vi "GET.series.vi"(4 "series offset":u32, 5 "request specific headers":T2[](array[typedef]), 6 "Number of Series to GET":u32, 7 "timeout (60000)":i32=60000, 8 "error in (no error)":errorcluster, 11 "REST Client in":refnum<class "REST Client.lvclass">) -> (0 "error out":errorcluster, 2 "data":T1, 3 "REST Client out":refnum<class "REST Client.lvclass">)   [LabVIEW 2024]
uses:
  <vilib>/addons/_JKI.lib/REST Client/classes/REST Client/HTTP Header.ctl
  <vilib>/NI/Advanced HTTP Client/Header--Combo Box.ctl
  <vilib>/addons/_JKI.lib/REST Client/classes/REST Client/REST Client.lvclass
  <vilib>/NI/Advanced HTTP Client/Session.lvclass
  TypeDefs/series.reply.ctl
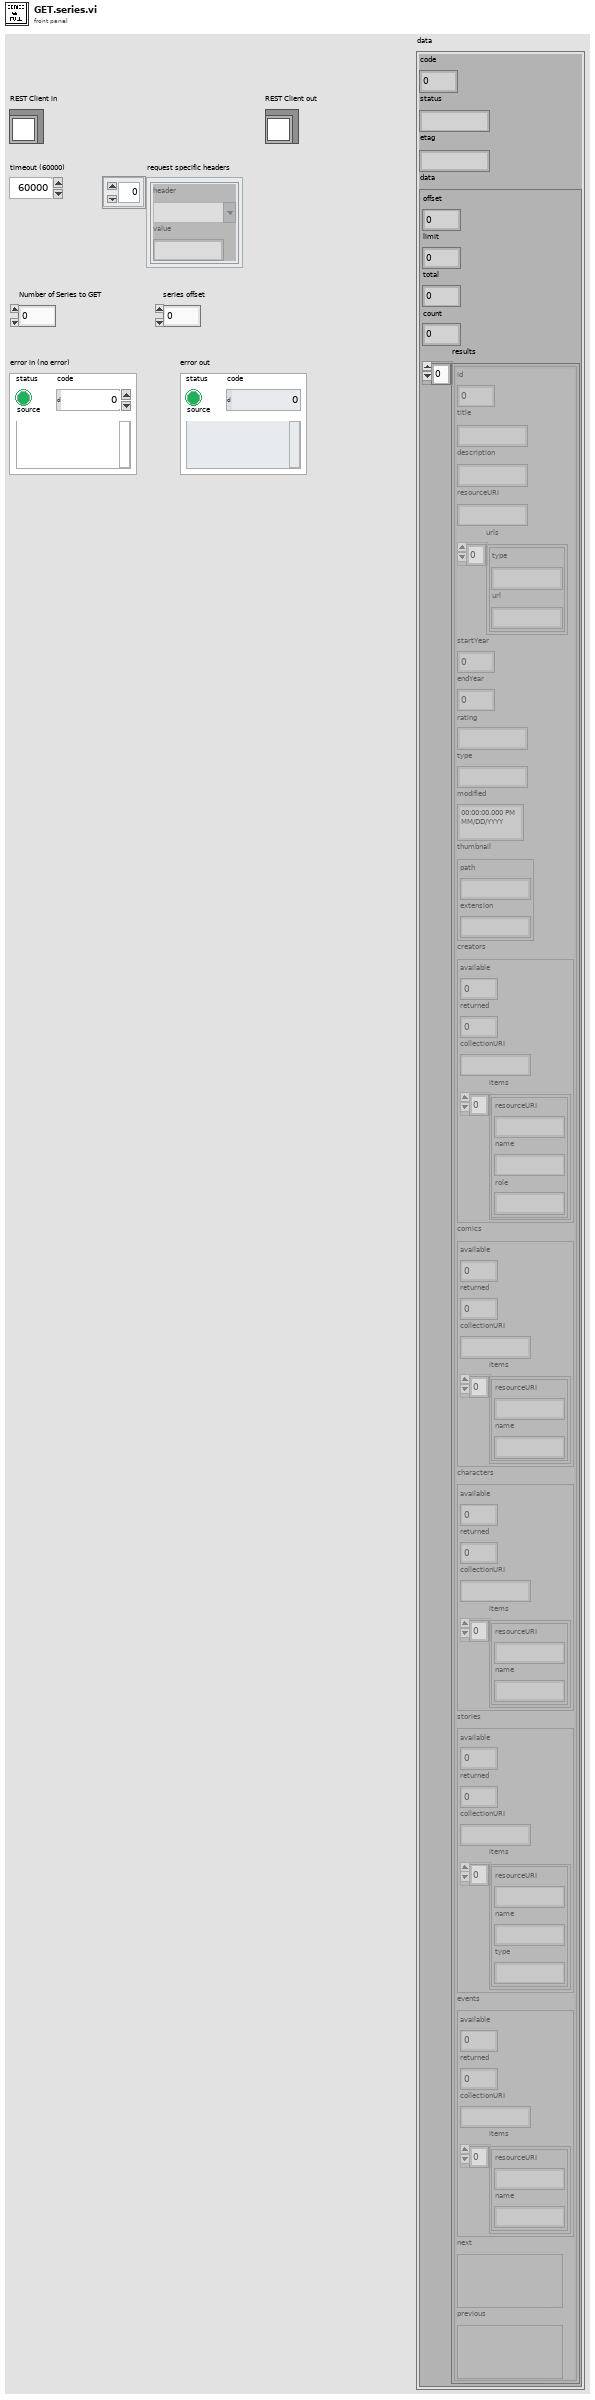
[diagram p1: front panel]
types:
  T1 = typedef "series.reply.ctl" = cluster{"code":i32, "status":string, "etag":string, "data":cluster{"offset":i32, "limit":i32, "total":i32, "count":i32, "results":cluster{"id":i32, "title":string, "description":string, "resourceURI":string, "urls":cluster{"type":string, "url":string}[], "startYear":i32, "endYear":i32, "rating":string, "type":string, "modified":timestamp, "thumbnail":cluster{"path":string, "extension":string}, "creators":cluster{"available":i32, "returned":i32, "collectionURI":string, "items":cluster{"resourceURI":string, "name":string, "role":string}[]}, "comics":cluster{"available":i32, "returned":i32, "collectionURI":string, "items":cluster{"resourceURI":string, "name":string}[]}, "characters":cluster{"available":i32, "returned":i32, "collectionURI":string, "items":cluster{"resourceURI":string, "name":string}[]}, "stories":cluster{"available":i32, "returned":i32, "collectionURI":string, "items":cluster{"resourceURI":string, "name":string, "type":string}[]}, "events":cluster{"available":i32, "returned":i32, "collectionURI":string, "items":cluster{"resourceURI":string, "name":string}[]}, "next":variant, "previous":variant}[]}}
  T2 = typedef "REST Client.lvlib/REST Client.lvclass/HTTP Header.ctl" = cluster{"header":T3, "value":string}
  T3 = typedef "lib_NI_Advanced HTTP Client.lvlib/Session.lvclass/Header--Combo Box.ctl" = string
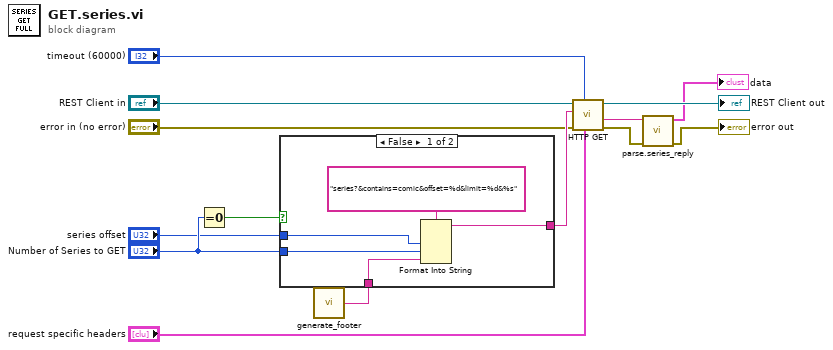
[diagram p0: block diagram]
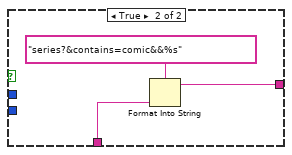
[diagram p2: hidden frame]
diagram:
  n1 = Equal To 0?(x="Number of Series to GET") -> (x = 0?=w2:bool)
  n2 = call "generate_footer.vi"() -> ("footer"=w9:string)  [unwired: 1 in]
  n3 = case shown="False" w2 {
    tunnel: [w19 w22] -> w10
    tunnel: w9 -> [w18 w20]
    tunnel: "series offset" -> [w17 _]
    tunnel: "Number of Series to GET" -> [w16 _]
    frame False {
      n4 = Format Into String(format string="series?&contains=comic&offset=%d&limit=%d&%s" ("Path"), w17, w16, w18) -> (resulting string=w19:string)  [unwired: 2 in, 1 out]
    }
    frame True {
      n5 = Format Into String(format string="series?&contains=comic&&%s" ("Path"), w20) -> (resulting string=w22:string)  [unwired: 2 in, 1 out]
    }
  }
  n6 = call-dynamic "HTTP GET.vi"("request specific headers"="request specific headers", "timeout (0 = Use Default)"="timeout (60000)", "error in (no error)"="error in (no error)", "Path"=w10, "REST Client in"="REST Client in") -> ("error out"=w12:errorcluster, "Response body"=w11:string, "REST Client out"=→"REST Client out":refnum<class "REST Client.lvclass">)  [unwired: 1 in, 3 out]
  n7 = call "parse.series_reply.vi"("error in"=w12, "string in"=w11) -> ("error out"=→"error out":errorcluster, "data"=→"data":T1)  [unwired: 8 in]
